vi "Serial_read.vi"(3 "error in (no error)":errorcluster, 4 "VISA resource name":refnum<visa-resource-name>, 5 "delay before read (ms)":u32) -> (0 "Response":string, 2 "bytes read":u32)   [LabVIEW 2018]
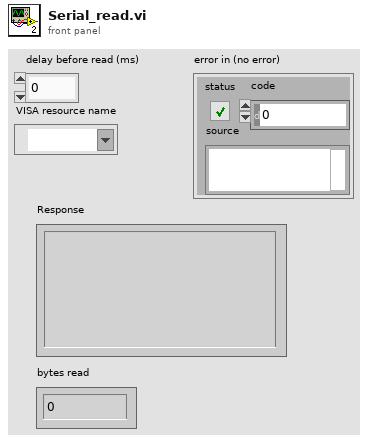
[diagram p1: front panel]
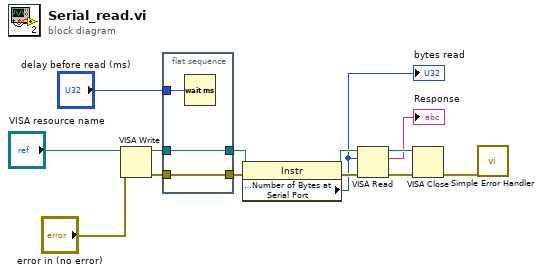
[diagram p0: block diagram]
diagram:
  n1 = VISA Write(VISA resource name="VISA resource name", error in (no error)="error in (no error)") -> (VISA resource name out=w9:refnum<visa-resource-name>, error out=w11:errorcluster)  [unwired: 1 in, 1 out]
  n2 = flat-sequence {
    tunnel: w11 -> [w16]
    tunnel: [w16] -> w10
    tunnel: w9 -> [w15]
    tunnel: [w15] -> w8
    tunnel: "delay before read (ms)" -> [w17]
    frame #0 {
      n3 = Wait (ms)(milliseconds to wait=w17) -> ()  [unwired: 1 out]
    }
  }
  n4 = property class="Instr"(reference=w8, error in=w10) -> (reference out=w7:refnum<visa-resource-name>, error out=w6:errorcluster, "Serial Settings:Number of Bytes at Serial Port"=w4:u32)
  "bytes read" <- w4
  n5 = VISA Read(VISA resource name=w7, byte count=w4, error in (no error)=w6) -> (VISA resource name out=w13:refnum<visa-resource-name>, read buffer=→"Response":string, error out=w14:errorcluster)  [unwired: 1 out]
  n6 = VISA Close(VISA resource name=w13, error in (no error)=w14) -> (error out=w12:errorcluster)
  n7 = call <vilib>:"Simple Error Handler.vi"("error in (no error)"=w12) -> ()  [unwired: 1 in, 8 out]
